vi "Read Voltage.vi"(8 "error in":errorcluster, 11 "Scope Base in":refnum<class "Scope Base.lvclass">) -> (0 "error out":errorcluster, 2 "Voltage":dbl format="%#_g V", 3 "Scope Base out":refnum<class "Scope Base.lvclass">)   [LabVIEW 2023, in "Scope.lvlib" / "Scope Base.lvlib" / "Scope Base.lvclass"]
uses:
  Scope Base.lvclass
  Interfaces/IConfigure Voltmeter/IConfigure Voltmeter.lvclass
  Scope Base.lvclass/Scope Base.ctl
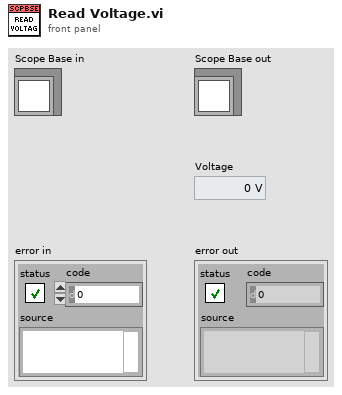
[diagram p1: front panel]
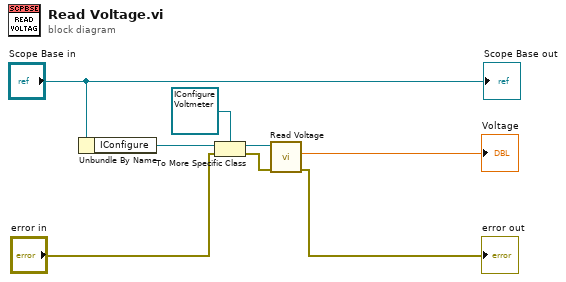
[diagram p0: block diagram]
diagram:
  n1 = Unbundle By Name("Scope Base in") -> ("IConfigure"=w1:refnum<class "IConfigure.lvclass">)
  n2 = To More Specific Class(target class=refnum<class "IConfigure Voltmeter.lvclass"> refnum ("IConfigure Voltmeter.lvclass"), reference=w1, error in="error in") -> (specific class reference=w7:refnum<class "IConfigure Voltmeter.lvclass">, error out=w6:errorcluster)
  n3 = call-dynamic "Read Voltage.vi"("error in"=w6, "IConfigure Voltmeter in"=w7) -> ("error out"=→"error out":errorcluster, "Voltage"=→"Voltage":dbl)  [unwired: 7 in, 1 out]
  "Scope Base out" <- "Scope Base in"
